vi "singleAxisMultiMove_MultiAxis.vi"(0 "Bd ID":T5=1 min=1 max=32 step=1, 1 "Axis":T3=1 items=["Axis Control"=0, "Axis 1"=1, "Axis 2"=2, "Axis 3"=3, "Axis 4"=4, "Axis 5"=5, "Axis 6"=6, "Axis 7"=7, "Axis 8"=8, "Vector Space Control"=16, "Vector Space 1"=17, "Vector Space 2"=18, "Vector Space 3"=19, "Vector Space 4"=20, "Encoder Control"=32, "Encoder 1"=33, "Encoder 2"=34, "Encoder 3"=35, "Encoder 4"=36, "Encoder 5"=37, "Encoder 6"=38, "Encoder 7"=39, "Encoder 8"=40, "DAC Channel 1"=49, "DAC Channel 2"=50, "DAC Channel 3"=51, "DAC Channel 4"=52, "DAC Channel 5"=53, "DAC Channel 6"=54, "DAC Channel 7"=55, "DAC Channel 8"=56, "Stepper Output 1"=65, "Stepper Output 2"=66, "Stepper Output 3"=67, "Stepper Output 4"=68, "Stepper Output 5"=69, "Stepper Output 6"=70, "Stepper Output 7"=71, "Stepper Output 8"=72, "ADC Channel 1"=81, "ADC Channel 2"=82, "ADC Channel 3"=83, "ADC Channel 4"=84, "ADC Channel 5"=85, "ADC Channel 6"=86, "ADC Channel 7"=87, "ADC Channel 8"=88], 5 "error in (no error)":errorcluster, 6 "Units (Encoder Counts)":T1=enum."Encoder Counts", 7 "Target Positions":dbl[](array[numeric]), 8 "Stop Refnum":refnum<vi>, 9 "Trajectory Parameters":T2={"Operation Mode (Absolute)"=0, "Blend"=FALSE, "Velocity"=6.0, "Acceleration"=4.0, "Deceleration"=4.0, "Blend Factor"=0, "Permitted Following Error"=1000.0, "S Curve Time"=0} {"Operation Mode (Absolute)" items=["Absolute Position", "Relative Position"]}) -> (14 "Bd ID Out":T4, 15 "Resource Output":T3 items=["Axis Control"=0, "Axis 1"=1, "Axis 2"=2, "Axis 3"=3, "Axis 4"=4, "Axis 5"=5, "Axis 6"=6, "Axis 7"=7, "Axis 8"=8, "Vector Space Control"=16, "Vector Space 1"=17, "Vector Space 2"=18, "Vector Space 3"=19, "Vector Space 4"=20, "Encoder Control"=32, "Encoder 1"=33, "Encoder 2"=34, "Encoder 3"=35, "Encoder 4"=36, "Encoder 5"=37, "Encoder 6"=38, "Encoder 7"=39, "Encoder 8"=40, "DAC Channel 1"=49, "DAC Channel 2"=50, "DAC Channel 3"=51, "DAC Channel 4"=52, "DAC Channel 5"=53, "DAC Channel 6"=54, "DAC Channel 7"=55, "DAC Channel 8"=56, "Stepper Output 1"=65, "Stepper Output 2"=66, "Stepper Output 3"=67, "Stepper Output 4"=68, "Stepper Output 5"=69, "Stepper Output 6"=70, "Stepper Output 7"=71, "Stepper Output 8"=72, "ADC Channel 1"=81, "ADC Channel 2"=82, "ADC Channel 3"=83, "ADC Channel 4"=84, "ADC Channel 5"=85, "ADC Channel 6"=86, "ADC Channel 7"=87, "ADC Channel 8"=88], 19 "error out":errorcluster)   [LabVIEW 2010]
doc: "Iterates through the passed in array of target positions on the given axis using the given trajectory parameters. Function exits when one of the following occurs:\n\n-All moves have been completed\n-A kill stop is performed on the axis\n-A true condition is detected on the control pointed to by Stop Refnum\n-An error condition is detected\n\nNotes:\n\nAll operations are done on the host computer (no buffering or onboard programming).\n\nUses the FlexMotion \"Load Target Position.flx\" to send target positions to the controller board."
uses:
  <vilib>/Motion/FlexMotion/CustomControls/CustomControls.llb/Resource Out (Enum).flx
  Shared/typedefs/Trajectory Parameters.ctl
  Typedefs/Units_Enum.ctl
  <vilib>/Motion/FlexMotion/FunctionsVIs/StartStopMotion.llb/Blend Motion (8 axes).flx
  <vilib>/Motion/FlexMotion/FunctionsVIs/StartStopMotion.llb/Start Motion (8 axes).flx
  <vilib>/Motion/FlexMotion/FunctionsVIs/Trajectory.llb/Check Blend Complete Status (8 axes).flx
  <vilib>/Motion/FlexMotion/FunctionsVIs/Trajectory.llb/Check Move Complete Status (8 axes).flx
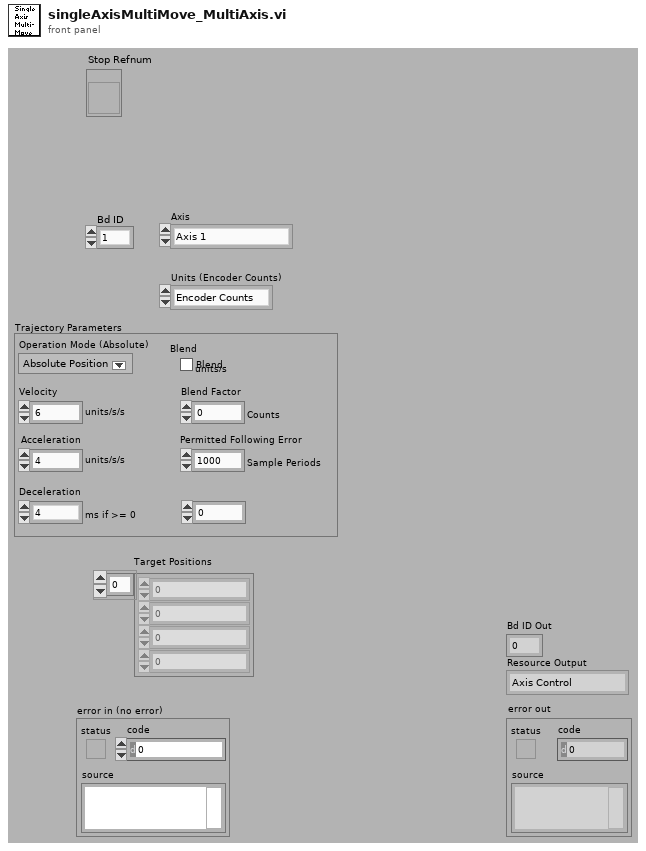
[diagram p1: front panel]
types:
  T1 = typedef "Units_Enum.ctl" = enum16{"Radians", "Encoder Counts", "Revolutions", "Degrees"}
  T2 = typedef "Trajectory Parameters.ctl" = cluster{"Operation Mode (Absolute)":u16, "Blend":bool, "Velocity":dbl, "Acceleration":dbl, "Deceleration":dbl, "Blend Factor":i16, "Permitted Following Error":dbl, "S Curve Time":u16}
  T3 = typedef "Resource Out (Enum).flx" = u16
  T4 = typedef "Bd Id Out" = u8
  T5 = typedef "Board Id" = u8
  T6 = cluster{"Run/Stop":bool, "Profile Complete":bool, "Motor Off ":bool, "Following Error":bool, "Limit Switch":bool, "Home Switch":bool, "SW Limit Switch":bool, "Watchdog":bool, "Velocity Threshold":bool, "Position Brkpt":bool, "Home Found":bool, "Index Found":bool, "High Speed Capture":bool, "Reverse Direction":bool, "Blend Complete":bool, "Move Complete":bool}
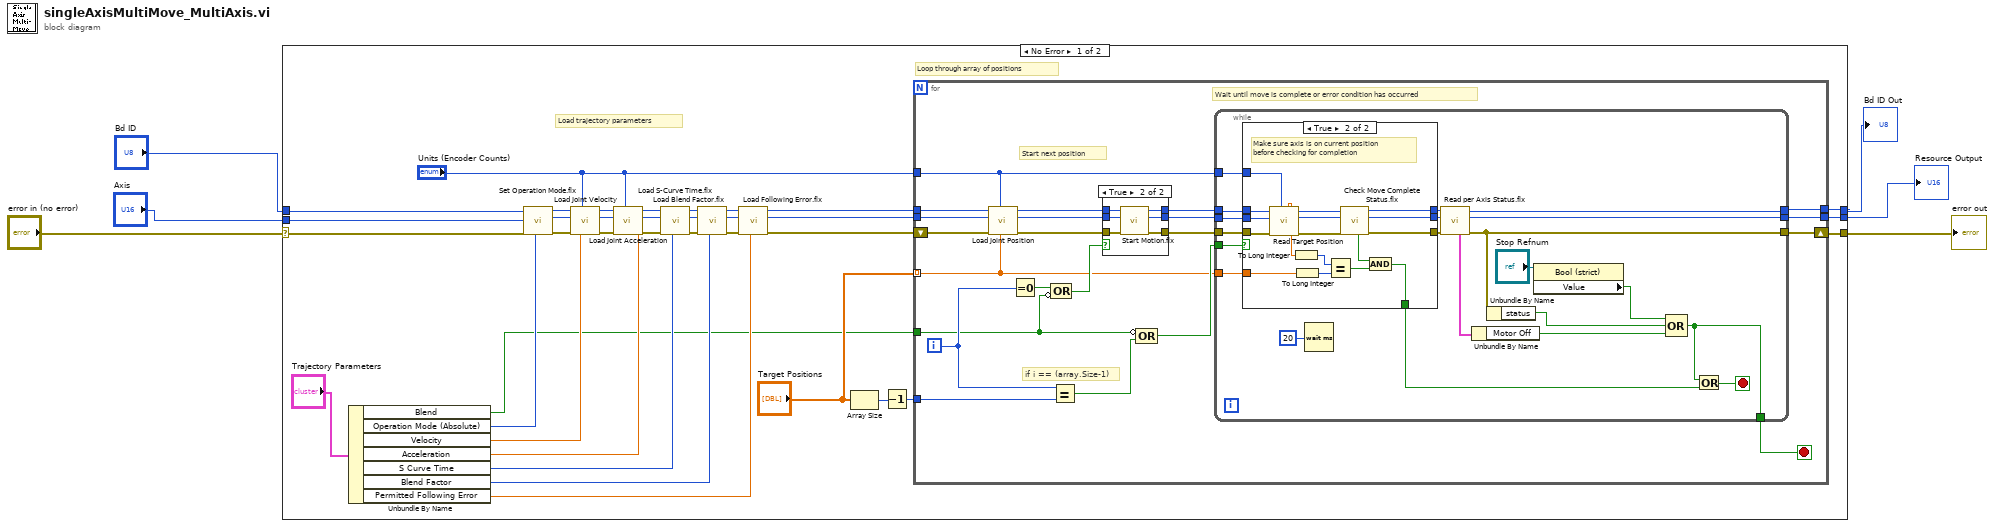
[diagram p0: block diagram]
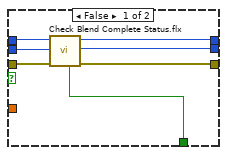
[diagram p2: hidden frame]
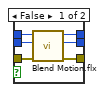
[diagram p3: hidden frame]
diagram:
  n1 = case shown="No Error" "error in (no error)" {
    selector: "error in (no error)" -> [w8 w122]
    tunnel: "Bd ID" -> [w42 w124]
    tunnel: "Axis" -> [w41 w123]
    tunnel: [w13 w122] -> w4
    tunnel: [w15 w123] -> w3
    tunnel: [w14 w124] -> w2
    frame No Error {
      # "Loop through array of positions"
      # "Load trajectory parameters"
      n2 = Unbundle By Name("Trajectory Parameters") -> ("Blend"=w7:bool, "Operation Mode (Absolute)"=w12:u16, "Velocity"=w22:dbl, "Acceleration"=w20:dbl, "S Curve Time"=w23:u16, "Blend Factor"=w16:i16, "Permitted Following Error"=w30:dbl)
      n3 = call <vilib>:"Set Operation Mode.flx"("Position Mode (Absolute)"=w12, "error in (no error)"=w8, "Axis or Vector Space"=w41, "Board ID"=w42) -> ("error out"=w38:errorcluster, "Resource Output"=w39:T3, "Bd ID Out"=w40:T4)  [unwired: 2 in]
      n4 = call "Load Joint Velocity.vi"("Units (Encoder Counts)"="Units (Encoder Counts)", "error in (no error)"=w38, "Velocity"=w22, "Axis"=w39, "Board ID"=w40) -> ("error out"=w19:errorcluster, "Resource Output"=w17:T3, "Bd ID Out"=w18:T4)  [unwired: 4 in]
      n5 = call "Load Joint Acceleration.vi"("Units (Encoder Counts)"="Units (Encoder Counts)", "error in (no error)"=w19, "Acceleration"=w20, "Axis"=w17, "Board ID"=w18) -> ("error out"=w24:errorcluster, "Resource Output"=w25:T3, "Bd ID Out"=w26:T4)  [unwired: 4 in]
      n6 = call <vilib>:"Load S-Curve Time.flx"("S Curve Time (1)"=w23, "error in (no error)"=w24, "Axis or Vector Space"=w25, "Board ID"=w26) -> ("error out"=w27:errorcluster, "Resource Output"=w28:T3, "Bd ID Out"=w29:T4)  [unwired: 3 in]
      n7 = call <vilib>:"Load Blend Factor.flx"("Blend Factor (-1)"=w16, "error in (no error)"=w27, "Axis or Vector Space"=w28, "Board ID"=w29) -> ("error out"=w37:errorcluster, "Resource Output"=w35:T3, "Bd ID Out"=w36:T4)  [unwired: 3 in]
      n8 = call <vilib>:"Load Following Error.flx"("Following Error"=w30, "error in (no error)"=w37, "Axis"=w35, "Board ID"=w36) -> ("error out"=w32:errorcluster, "Resource Output"=w33:T3, "Bd ID Out"=w34:T4)  [unwired: 3 in]
      n9 = Array Size(array="Target Positions") -> (size(s)=w9:i32)
      n10 = Decrement(x=w9) -> (x-1=w10:i32)
      n11 = for {
        shift-left: w32 -> [w59]
        shift-right: [w48] -> w13
        tunnel: "Target Positions" -> [w47] mode=indexing
        tunnel: w10 -> [w44]
        tunnel: w33 -> [w61]
        tunnel: w34 -> [w60]
        tunnel: [w49] -> w15
        tunnel: [w50] -> w14
        tunnel: "Units (Encoder Counts)" -> [w45]
        tunnel: w7 -> [w43]
        i -> [w53]
        stop <- w46 stop-if-true
        # "Start next position"
        # "if i == (array.Size-1)"
        # "Wait until move is complete or error condition has occurred"
        n12 = call "Load Joint Position.vi"("Units (Encoder Counts)"=w45, "error in (no error)"=w59, "Target Position"=w47, "Axis"=w61, "Board ID"=w60) -> ("error out"=w62:errorcluster, "Resource Output"=w63:T3, "Bd ID Out"=w64:T4)  [unwired: 4 in]
        n13 = Equal To 0?(x=w53) -> (x = 0?=w52:bool)
        n14 = Compound Arithmetic op=OR(w52, invert w43) -> (w58:bool)
        n15 = Equal?(x=w53, y=w44) -> (x = y?=w57:bool)
        n16 = case shown="True" w58 {
          tunnel: w64 -> [w115 w121]
          tunnel: w63 -> [w114 w120]
          tunnel: w62 -> [w113 w119]
          tunnel: [w112 w118] -> w56
          tunnel: [w111 w117] -> w55
          tunnel: [w110 w116] -> w54
          frame False {
            n17 = call-poly <vilib>:"Blend Motion.flx"("error in (no error)"=w113, "Axis or Vector Space"=w114, "Board ID"=w115) -> ("error out"=w110:errorcluster, "Resource Output"=w111:T3, "Bd ID Out"=w112:T4)  [unwired: 3 in]
          }
          frame True {
            n18 = call-poly <vilib>:"Start Motion.flx"("error in (no error)"=w119, "Axis or Vector Space"=w120, "Board ID"=w121) -> ("error out"=w116:errorcluster, "Resource Output"=w117:T3, "Bd ID Out"=w118:T4)  [unwired: 3 in]
          }
        }
        n19 = Compound Arithmetic op=OR(invert w43, w57) -> (w51:bool)
        n20 = while {
          tunnel: w56 -> [w72]
          tunnel: w55 -> [w71]
          tunnel: w54 -> [w70]
          tunnel: [w77] -> w48
          tunnel: [w80] -> w49
          tunnel: [w81] -> w50
          tunnel: [w73] -> w46
          tunnel: w51 -> [w69]
          tunnel: w47 -> [w68]
          tunnel: w45 -> [w67]
          stop <- w84 stop-if-true
          n21 = case shown="True" w69 {
            tunnel: w70 -> [w90 w104]
            tunnel: w71 -> [w91 w105]
            tunnel: w72 -> [w92 w106]
            tunnel: [w89 w107] -> w82
            tunnel: [w87 w109] -> w79
            tunnel: [w88 w108] -> w78
            tunnel: [w86 w100] -> w74
            tunnel: w68 -> [_ w95]
            tunnel: w67 -> [_ w97]
            frame False {
              n22 = call-poly <vilib>:"Check Blend Complete Status.flx"("error in (no error)"=w90, "Axis or Vector Space"=w91, "Board ID"=w92) -> ("error out"=w89:errorcluster, "Resource Output"=w88:T3, "Bd ID Out"=w87:T4, "Blend Complete"=w86:bool)  [unwired: 3 in]
            }
            frame True {
              # "Make sure axis is on current position\nbefore checking for completion"
              n23 = call "Read Target Position.vi"("Units (Encoder Counts)"=w97, "error in (no error)"=w104, "Axis"=w105, "Board ID"=w106) -> ("error out"=w103:errorcluster, "Resource Output"=w102:T3, "Bd ID Out"=w101:T4, "Target Position"=w93:dbl)  [unwired: 4 in]
              n24 = To Long Integer(number=w93) -> (32bit integer=w96:i32)
              n25 = To Long Integer(number=w95) -> (32bit integer=w94:i32)
              n26 = Equal?(x=w96, y=w94) -> (x = y?=w99:bool)
              n27 = call-poly <vilib>:"Check Move Complete Status.flx"("error in (no error)"=w103, "Axis or Vector Space"=w102, "Board ID"=w101) -> ("error out"=w107:errorcluster, "Resource Output"=w108:T3, "Bd ID Out"=w109:T4, "Move Complete"=w98:bool)  [unwired: 3 in]
              n28 = And(x=w98, y=w99) -> (x .and. y?=w100:bool)
            }
          }
          n29 = Wait (ms)(milliseconds to wait=u32 20) -> ()  [unwired: 1 out]
          n30 = call <vilib>:"Read per Axis Status.flx"("error in (no error)"=w82, "Axis"=w78, "Board ID"=w79) -> ("error out"=w77:errorcluster, "Resource Output"=w80:T3, "Bd ID Out"=w81:T4, "Per Axis H/W Status"=w85:T6)  [unwired: 3 in]
          n31 = Unbundle By Name(w85) -> ("Motor Off"=w76:bool)
          n32 = Unbundle By Name(w77) -> ("status"=w75:bool)
          n33 = property class="Bool (strict)"(reference="Stop Refnum") -> ("Value"=w65:bool)  [unwired: 1 in, 2 out]
          n34 = Compound Arithmetic op=OR(w65, w75, w76) -> (w73:bool)
          n35 = Or(x=w73, y=w74) -> (x .or. y?=w84:bool)
        }
      }
    }
    frame Error {
    }
  }
  "error out" <- w4
  "Bd ID Out" <- w2
  "Resource Output" <- w3
